vi "GatherSpinParameter.vi"(2 "路径":path) -> (0 "ProgressFinalSpin":T4, 1 "FinalSpinEnd_Index":u32, 3 "RUNStateID":T1, 4 "EXCEL读取":string[][](array[string]), 5 "ProgressInitial":T3, 6 "POWERStateID":T2)   [LabVIEW 2011]
panel:
  # "常用参数：\nPogress_FinalSpin_Index:  用于存储PogressFinalSpinIndex, 用于标定\nFinalSpin_SetpDrain: 用于存储SepDain, 标定\nFinalSpin_StepSpin: 用于活动Spin阶段，进行时间比较\nFinalSpin_StepLoose: 用于活动Loose阶段，标定，而后开始比较"
  # "常用参数：\nPOWER_UPSTGART_Index： 整机正在上电\nPOWER_ON_Idex： 整机处于完全上电状态"
  # "常用参数：\nInitial_StepFirstDrain,(用于计算差价)"
  # "常用参数：\nRUNMODE_READY_Index : 整机准备运行状态\nRUNMODE_RUNNING_Index : 整机处于运行状态"
  # "常用参数：\nFinalSpinEnd_Index: 用于表示数据比对结束"
  # "Useful"
  # "Useful"
  # "Useful"
  # "Useful"
  # "Useful"
  # "Useful"
  # "Useful"
  # "Useful"
  # "Useful"
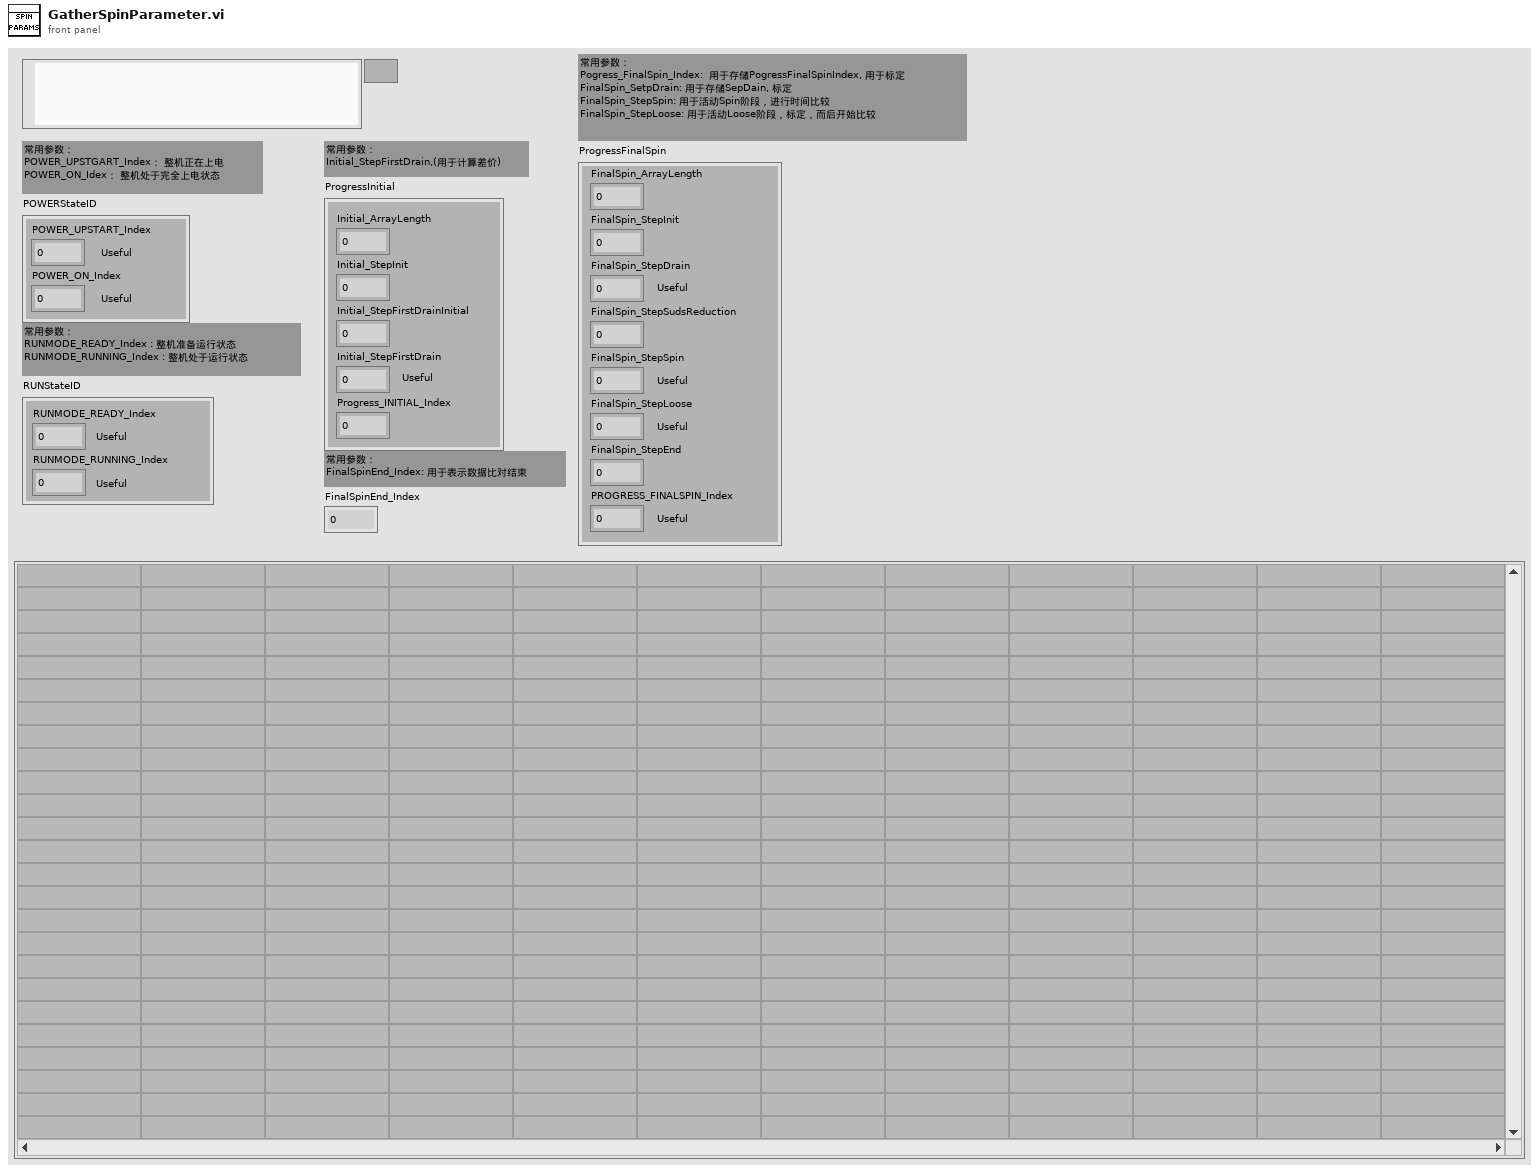
[diagram p1: front panel]
types:
  T1 = cluster{"RUNMODE_READY_Index":u32, "RUNMODE_RUNNING_Index":u32}
  T2 = cluster{"POWER_UPSTART_Index":u32, "POWER_ON_Index":u32}
  T3 = cluster{"Initial_ArrayLength":u32, "Initial_StepInit":u32, "Initial_StepFirstDrainInitial":u32, "Initial_StepFirstDrain":u32, "Progress_INITIAL_Index":u32}
  T4 = cluster{"FinalSpin_ArrayLength":u32, "FinalSpin_StepInit":u32, "FinalSpin_StepDrain":u32, "FinalSpin_StepSudsReduction":u32, "FinalSpin_StepSpin":u32, "FinalSpin_StepLoose":u32, "FinalSpin_StepEnd":u32, "PROGRESS_FINALSPIN_Index":u32}
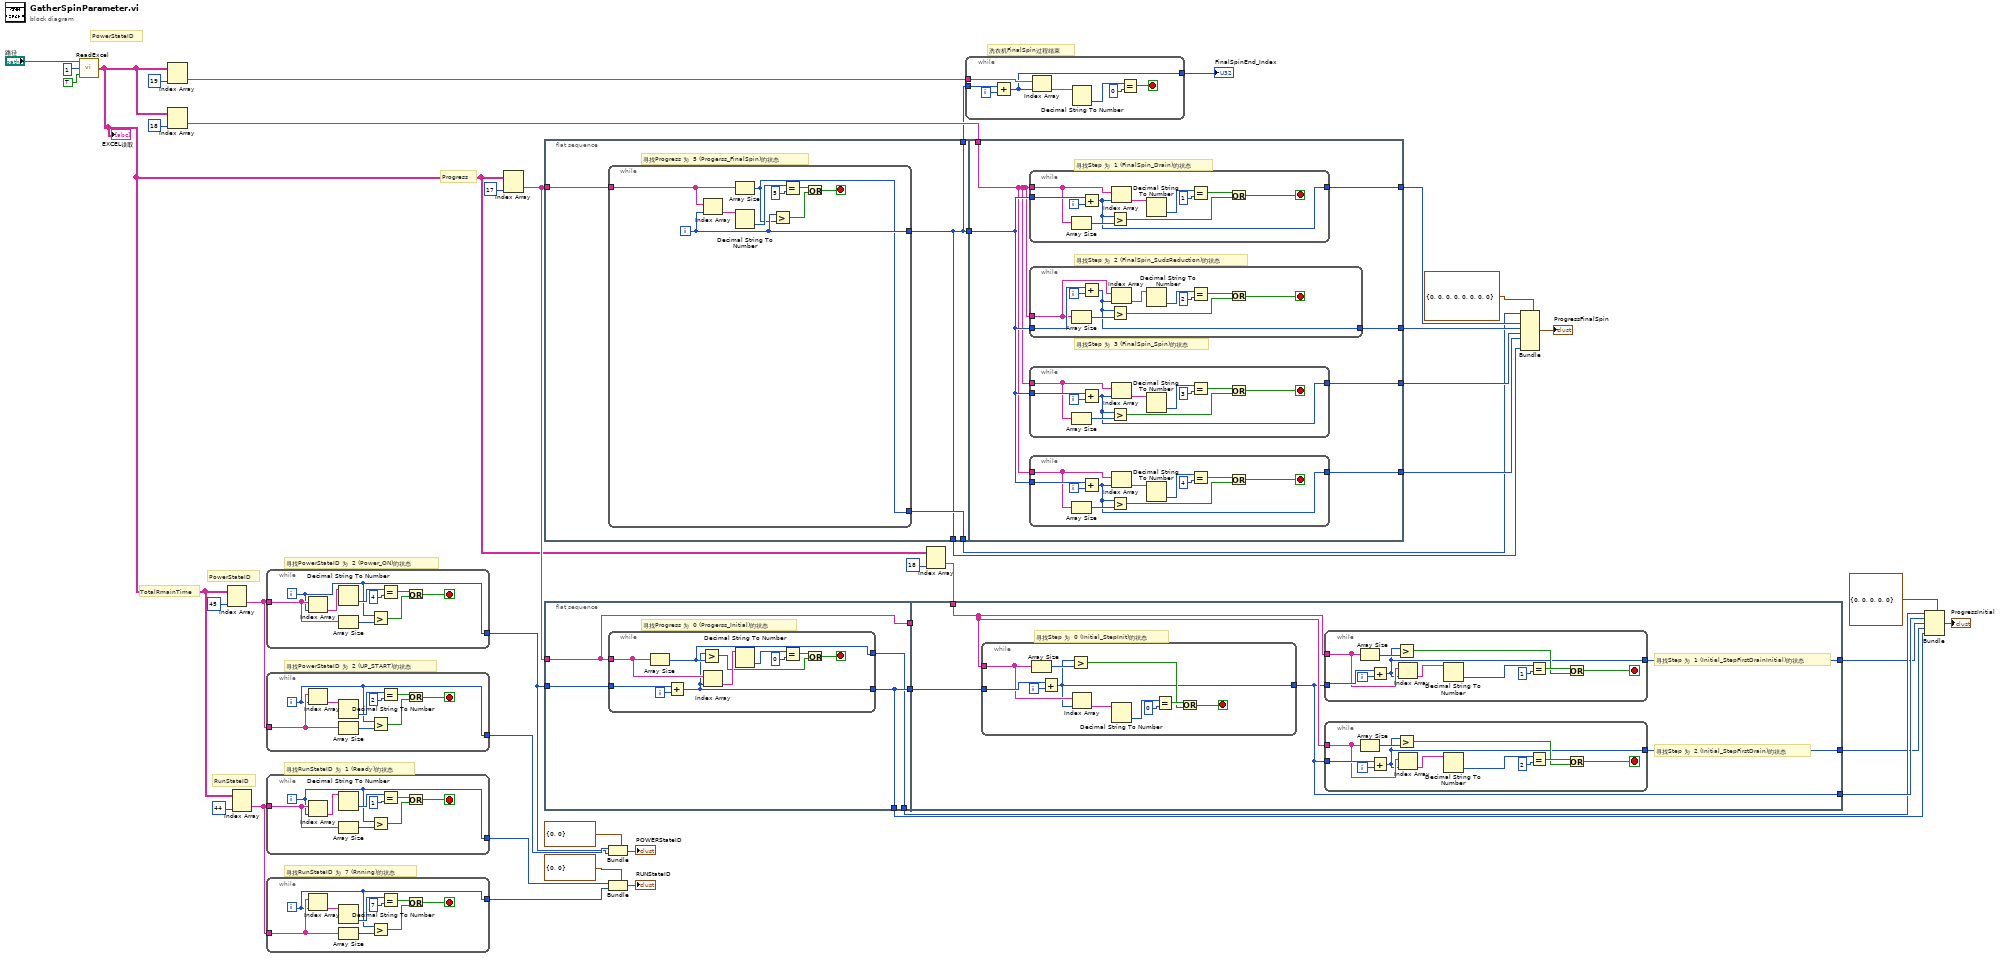
[diagram p0: block diagram]
diagram:
  # "PowerStateID"
  # "TotalRmainTime"
  # "洗衣机FinalSpin过程结束"
  # "Progress"
  # "PowerStateID"
  # "RunStateID"
  # "寻找PowerStateID 为  2 (Power_ON)的状态"
  # "寻找PowerStateID 为  2 (UP_START)的状态"
  # "寻找RunStateID 为  1 (Ready)的状态"
  # "寻找RunStateID 为  7 (Rnning)的状态"
  n1 = call "ReadExcel.vi"("读出文本"=TRUE, "导出sheet位号"=i8 1, "路径"="路径") -> ("EXCEL读取"=w13:string[][])
  "EXCEL读取" <- w13
  n2 = Index Array(array=w13, index (col)=19 ("禁用的索引 (列)")) -> (element=w11:string[])  [unwired: 1 in]
  n3 = Index Array(array=w13, index (col)=18 ("禁用的索引 (列)")) -> (element=w34:string[])  [unwired: 1 in]
  n4 = Index Array(array=w13, index (col)=45 ("索引 (行)")) -> (element=w38:string[])  [unwired: 1 in]
  n5 = Index Array(array=w13, index (col)=44 ("索引 (行)")) -> (element=w40:string[])  [unwired: 1 in]
  n6 = while {
    tunnel: w38 -> [w51]
    tunnel: [w49] -> w1
    i -> [w49]
    stop <- w45 stop-if-true
    n7 = Index Array(array=w51, index=w49) -> (element=w53:string)
    n8 = Decimal String To Number(string=w53) -> (number=w52:i32)  [unwired: 2 in, 1 out]
    n9 = Array Size(array=w51) -> (size(s)=w48:i32)
    n10 = Greater?(x=w49, y=w48) -> (0:w46:bool)
    n11 = Equal?(x=w52, y=4) -> (x = y?=w47:bool)
    n12 = Or(x=w47, y=w46) -> (x .or. y?=w45:bool)
  }
  n13 = while {
    tunnel: w38 -> [w60]
    tunnel: [w58] -> w7
    i -> [w58]
    stop <- w54 stop-if-true
    n14 = Index Array(array=w60, index=w58) -> (element=w62:string)
    n15 = Decimal String To Number(string=w62) -> (number=w61:i32)  [unwired: 2 in, 1 out]
    n16 = Array Size(array=w60) -> (size(s)=w57:i32)
    n17 = Greater?(x=w58, y=w57) -> (0:w55:bool)
    n18 = Equal?(x=w61, y=2) -> (x = y?=w56:bool)
    n19 = Or(x=w56, y=w55) -> (x .or. y?=w54:bool)
  }
  n20 = while {
    tunnel: w40 -> [w69]
    tunnel: [w67] -> w3
    i -> [w67]
    stop <- w63 stop-if-true
    n21 = Index Array(array=w69, index=w67) -> (element=w71:string)
    n22 = Decimal String To Number(string=w71) -> (number=w70:i32)  [unwired: 2 in, 1 out]
    n23 = Array Size(array=w69) -> (size(s)=w66:i32)
    n24 = Greater?(x=w67, y=w66) -> (0:w64:bool)
    n25 = Equal?(x=w70, y=1) -> (x = y?=w65:bool)
    n26 = Or(x=w65, y=w64) -> (x .or. y?=w63:bool)
  }
  n27 = while {
    tunnel: w40 -> [w78]
    tunnel: [w76] -> w2
    i -> [w76]
    stop <- w72 stop-if-true
    n28 = Index Array(array=w78, index=w76) -> (element=w80:string)
    n29 = Decimal String To Number(string=w80) -> (number=w79:i32)  [unwired: 2 in, 1 out]
    n30 = Array Size(array=w78) -> (size(s)=w75:i32)
    n31 = Greater?(x=w76, y=w75) -> (0:w73:bool)
    n32 = Equal?(x=w79, y=7) -> (x = y?=w74:bool)
    n33 = Or(x=w74, y=w73) -> (x .or. y?=w72:bool)
  }
  n34 = Index Array(array=w13, index (col)=17 ("禁用的索引 (列)")) -> (element=w23:string[])  [unwired: 1 in]
  n35 = flat-sequence {
    tunnel: w23 -> [w83]
    tunnel: [w81] -> w36
    tunnel: [w81] -> w27
    tunnel: [w82] -> w26
    tunnel: [w81] -> w10
    tunnel: w36 -> [w95]
    tunnel: w34 -> [w94]
    tunnel: [w98] -> w32
    tunnel: [w97] -> w31
    tunnel: [w96] -> w30
    tunnel: [w93] -> w29
    frame #0 {
      # "寻找Progress 为  5 (Progerss_FinalSpin)的状态"
      n36 = while {
        tunnel: w83 -> [w89]
        tunnel: [w85] -> w81
        tunnel: [w84] -> w82
        i -> [w85]
        stop <- w86 stop-if-true
        n37 = Index Array(array=w89, index=w85) -> (element=w92:string)
        n38 = Array Size(array=w89) -> (size(s)=w84:i32)
        n39 = Decimal String To Number(string=w92) -> (number=w91:i32)  [unwired: 2 in, 1 out]
        n40 = Greater?(x=w85, y=w84) -> (0:w87:bool)
        n41 = Equal?(x=w91, y=5) -> (x = y?=w88:bool)
        n42 = Or(x=w88, y=w87) -> (x .or. y?=w86:bool)
      }
    }
    frame #1 {
      # "寻找Step 为  3 (FinalSpin_Spin)的状态"
      # "寻找Step 为  2 (FinalSpin_SudsReduction)的状态"
      # "寻找Step 为  1 (FinalSpin_Drain)的状态"
      n43 = while {
        tunnel: w95 -> [w142]
        tunnel: w94 -> [w132]
        tunnel: [w133] -> w98
        i -> [w141]
        stop <- w134 stop-if-true
        n44 = Array Size(array=w132) -> (size(s)=w137:i32)
        n45 = Add(x=w142, y=w141) -> (x+y=w133:i32)
        n46 = Greater?(x=w133, y=w137) -> (0:w135:bool)
        n47 = Index Array(array=w132, index=w133) -> (element=w140:string)
        n48 = Decimal String To Number(string=w140) -> (number=w139:i32)  [unwired: 2 in, 1 out]
        n49 = Equal?(x=w139, y=1) -> (x = y?=w136:bool)
        n50 = Or(x=w136, y=w135) -> (x .or. y?=w134:bool)
      }
      n51 = while {
        tunnel: w95 -> [w131]
        tunnel: w94 -> [w121]
        tunnel: [w122] -> w97
        i -> [w130]
        stop <- w123 stop-if-true
        n52 = Array Size(array=w121) -> (size(s)=w126:i32)
        n53 = Add(x=w131, y=w130) -> (x+y=w122:i32)
        n54 = Greater?(x=w122, y=w126) -> (0:w124:bool)
        n55 = Index Array(array=w121, index=w122) -> (element=w129:string)
        n56 = Decimal String To Number(string=w129) -> (number=w128:i32)  [unwired: 2 in, 1 out]
        n57 = Equal?(x=w128, y=2) -> (x = y?=w125:bool)
        n58 = Or(x=w125, y=w124) -> (x .or. y?=w123:bool)
      }
      n59 = while {
        tunnel: w95 -> [w120]
        tunnel: w94 -> [w110]
        tunnel: [w111] -> w96
        i -> [w119]
        stop <- w112 stop-if-true
        n60 = Array Size(array=w110) -> (size(s)=w115:i32)
        n61 = Add(x=w120, y=w119) -> (x+y=w111:i32)
        n62 = Greater?(x=w111, y=w115) -> (0:w113:bool)
        n63 = Index Array(array=w110, index=w111) -> (element=w118:string)
        n64 = Decimal String To Number(string=w118) -> (number=w117:i32)  [unwired: 2 in, 1 out]
        n65 = Equal?(x=w117, y=3) -> (x = y?=w114:bool)
        n66 = Or(x=w114, y=w113) -> (x .or. y?=w112:bool)
      }
      n67 = while {
        tunnel: w95 -> [w109]
        tunnel: w94 -> [w99]
        tunnel: [w100] -> w93
        i -> [w108]
        stop <- w101 stop-if-true
        n68 = Array Size(array=w99) -> (size(s)=w104:i32)
        n69 = Add(x=w109, y=w108) -> (x+y=w100:i32)
        n70 = Greater?(x=w100, y=w104) -> (0:w102:bool)
        n71 = Index Array(array=w99, index=w100) -> (element=w107:string)
        n72 = Decimal String To Number(string=w107) -> (number=w106:i32)  [unwired: 2 in, 1 out]
        n73 = Equal?(x=w106, y=4) -> (x = y?=w103:bool)
        n74 = Or(x=w103, y=w102) -> (x .or. y?=w101:bool)
      }
    }
  }
  n75 = flat-sequence {
    tunnel: w23 -> [w145]
    tunnel: [w146] -> w20
    tunnel: [w146] -> w22
    tunnel: [w145] -> w21
    tunnel: [w144] -> w18
    tunnel: w1 -> [w143]
    tunnel: w22 -> [w162]
    tunnel: w21 -> [_]
    tunnel: [w158] -> w19
    tunnel: [w161] -> w17
    tunnel: [w160] -> w16
    tunnel: w14 -> [w159]
    frame #0 {
      # "寻找Progress 为  0 (Progerss_Initial)的状态"
      n76 = while {
        tunnel: w145 -> [w154]
        tunnel: [w148] -> w146
        tunnel: [w150] -> w144
        tunnel: w143 -> [w147]
        i -> [w149]
        stop <- w151 stop-if-true
        n77 = Array Size(array=w154) -> (size(s)=w150:i32)
        n78 = Add(x=w147, y=w149) -> (x+y=w148:i32)
        n79 = Greater?(x=w148, y=w150) -> (0:w152:bool)
        n80 = Index Array(array=w154, index=w148) -> (element=w157:string)
        n81 = Decimal String To Number(string=w157) -> (number=w156:i32)  [unwired: 2 in, 1 out]
        n82 = Equal?(x=w156, y=0) -> (x = y?=w153:bool)
        n83 = Or(x=w153, y=w152) -> (x .or. y?=w151:bool)
      }
    }
    frame #1 {
      # "寻找Step 为  2 (Initial_StepFirstDrain)的状态"
      # "寻找Step 为  1 (Initial_StepFirstDrainInitial)的状态"
      # "寻找Step 为  0 (Initial_StepInit)的状态"
      n84 = while {
        tunnel: w162 -> [w195]
        tunnel: w159 -> [w186]
        tunnel: [w185] -> w158
        i -> [w194]
        stop <- w187 stop-if-true
        n85 = Array Size(array=w186) -> (size(s)=w190:i32)
        n86 = Add(x=w195, y=w194) -> (x+y=w185:i32)
        n87 = Greater?(x=w185, y=w190) -> (0:w188:bool)
        n88 = Index Array(array=w186, index=w185) -> (element=w193:string)
        n89 = Decimal String To Number(string=w193) -> (number=w192:i32)  [unwired: 2 in, 1 out]
        n90 = Equal?(x=w192, y=0) -> (x = y?=w189:bool)
        n91 = Or(x=w189, y=w188) -> (x .or. y?=w187:bool)
      }
      n92 = while {
        tunnel: w158 -> [w184]
        tunnel: w159 -> [w175]
        tunnel: [w174] -> w161
        i -> [w183]
        stop <- w176 stop-if-true
        n93 = Array Size(array=w175) -> (size(s)=w179:i32)
        n94 = Add(x=w184, y=w183) -> (x+y=w174:i32)
        n95 = Greater?(x=w174, y=w179) -> (0:w177:bool)
        n96 = Index Array(array=w175, index=w174) -> (element=w182:string)
        n97 = Decimal String To Number(string=w182) -> (number=w181:i32)  [unwired: 2 in, 1 out]
        n98 = Equal?(x=w181, y=1) -> (x = y?=w178:bool)
        n99 = Or(x=w178, y=w177) -> (x .or. y?=w176:bool)
      }
      n100 = while {
        tunnel: w158 -> [w173]
        tunnel: w159 -> [w164]
        tunnel: [w163] -> w160
        i -> [w172]
        stop <- w165 stop-if-true
        n101 = Array Size(array=w164) -> (size(s)=w168:i32)
        n102 = Add(x=w173, y=w172) -> (x+y=w163:i32)
        n103 = Greater?(x=w163, y=w168) -> (0:w166:bool)
        n104 = Index Array(array=w164, index=w163) -> (element=w171:string)
        n105 = Decimal String To Number(string=w171) -> (number=w170:i32)  [unwired: 2 in, 1 out]
        n106 = Equal?(x=w170, y=2) -> (x = y?=w167:bool)
        n107 = Or(x=w167, y=w166) -> (x .or. y?=w165:bool)
      }
    }
  }
  n108 = Bundle(cluster=cluster{u32, u32} {0, 0}, w7, w1) -> (→"POWERStateID":cluster{u32, u32})
  n109 = Bundle(cluster=cluster{u32, u32} {0, 0}, w3, w2) -> (→"RUNStateID":cluster{u32, u32})
  n110 = Index Array(array=w13, index (col)=18 ("禁用的索引 (列)")) -> (element=w14:string[])  [unwired: 1 in]
  n111 = while {
    tunnel: w11 -> [w203]
    tunnel: w10 -> [w201]
    tunnel: [w196] -> w9
    i -> [w202]
    stop <- w197 stop-if-true
    n112 = Add(x=w201, y=w202) -> (x+y=w196:i32)
    n113 = Index Array(array=w203, index=w196) -> (element=w200:string)
    n114 = Decimal String To Number(string=w200) -> (number=w199:i32)  [unwired: 2 in, 1 out]
    n115 = Equal?(x=w199, y=0) -> (x = y?=w197:bool)
  }
  "FinalSpinEnd_Index" <- w9
  n116 = Bundle(cluster=cluster{u32, u32, u32, u32, u32, u32, u32, u32} {0, 0, 0, 0, 0, 0, 0, 0}, w26, w32, w31, w30, w29, w27) -> (→"ProgressFinalSpin":cluster{u32, u32, u32, u32, u32, u32, u32, u32})  [unwired: 2 in]
  n117 = Bundle(cluster=cluster{u32, u32, u32, u32, u32} {0, 0, 0, 0, 0}, w18, w19, w17, w16, w20) -> (→"ProgressInitial":cluster{u32, u32, u32, u32, u32})
